vi "e.gate HighSpeedPort Diagnostics Internal.vi"(0 "e.gate Configuration":T1 {"StartTime" format="%#.10f"; "dActTimeToSecondFactor" format="%#.10f"; "StartTimeToDayFactor" format="%#_10f"}, 11 "error in (no error)":errorcluster) -> (4 "e.gate Configuration out":T1 {"StartTime" format="%#.10f"; "dActTimeToSecondFactor" format="%#.10f"; "StartTimeToDayFactor" format="%#_10f"}, 6 "e.gate Interface Diagnostic Data":T9={"Interface Kind"=["Fieldbus", "Internal System", "Internal System", "ExternalUART", "ExternalUART", "ExternalUART"], "Interface Index"=[0, 0, 0, 0, 1, 2], "Cycles Count"=[280401, 280401, 280401, 280401, 14024, 280401], "Error Count"=[0, 0, 0, 0, 0, 0], "DeltaTimeS"=[1402.004973, 1402.004982, 1402.004982, 1402.004982, 1402.004983, 1402.004983]}, 8 "e.gate Transport Diagnostic Data":T8, 10 "e.gate Variable Diagnostic Data":T7, 15 "error out":errorcluster)   [LabVIEW 2016]
uses:
  e.gate Diagnostic Interface Data.ctl
  e.gate Diagnostic Transport Data.ctl
  e.gate Diagnostic Variable Data.ctl
  e.gate Configuration.ctl
  e.gate Channel Data.ctl
  e.gate Data Type.ctl
  e.gate Protocol Type.ctl
  e.gate Module  Data.ctl
  e.gateHSP_DLLhandle.ctl
panel:
  out "Structure ID":i8
  out "Remaining Data":u8[](array[numeric])
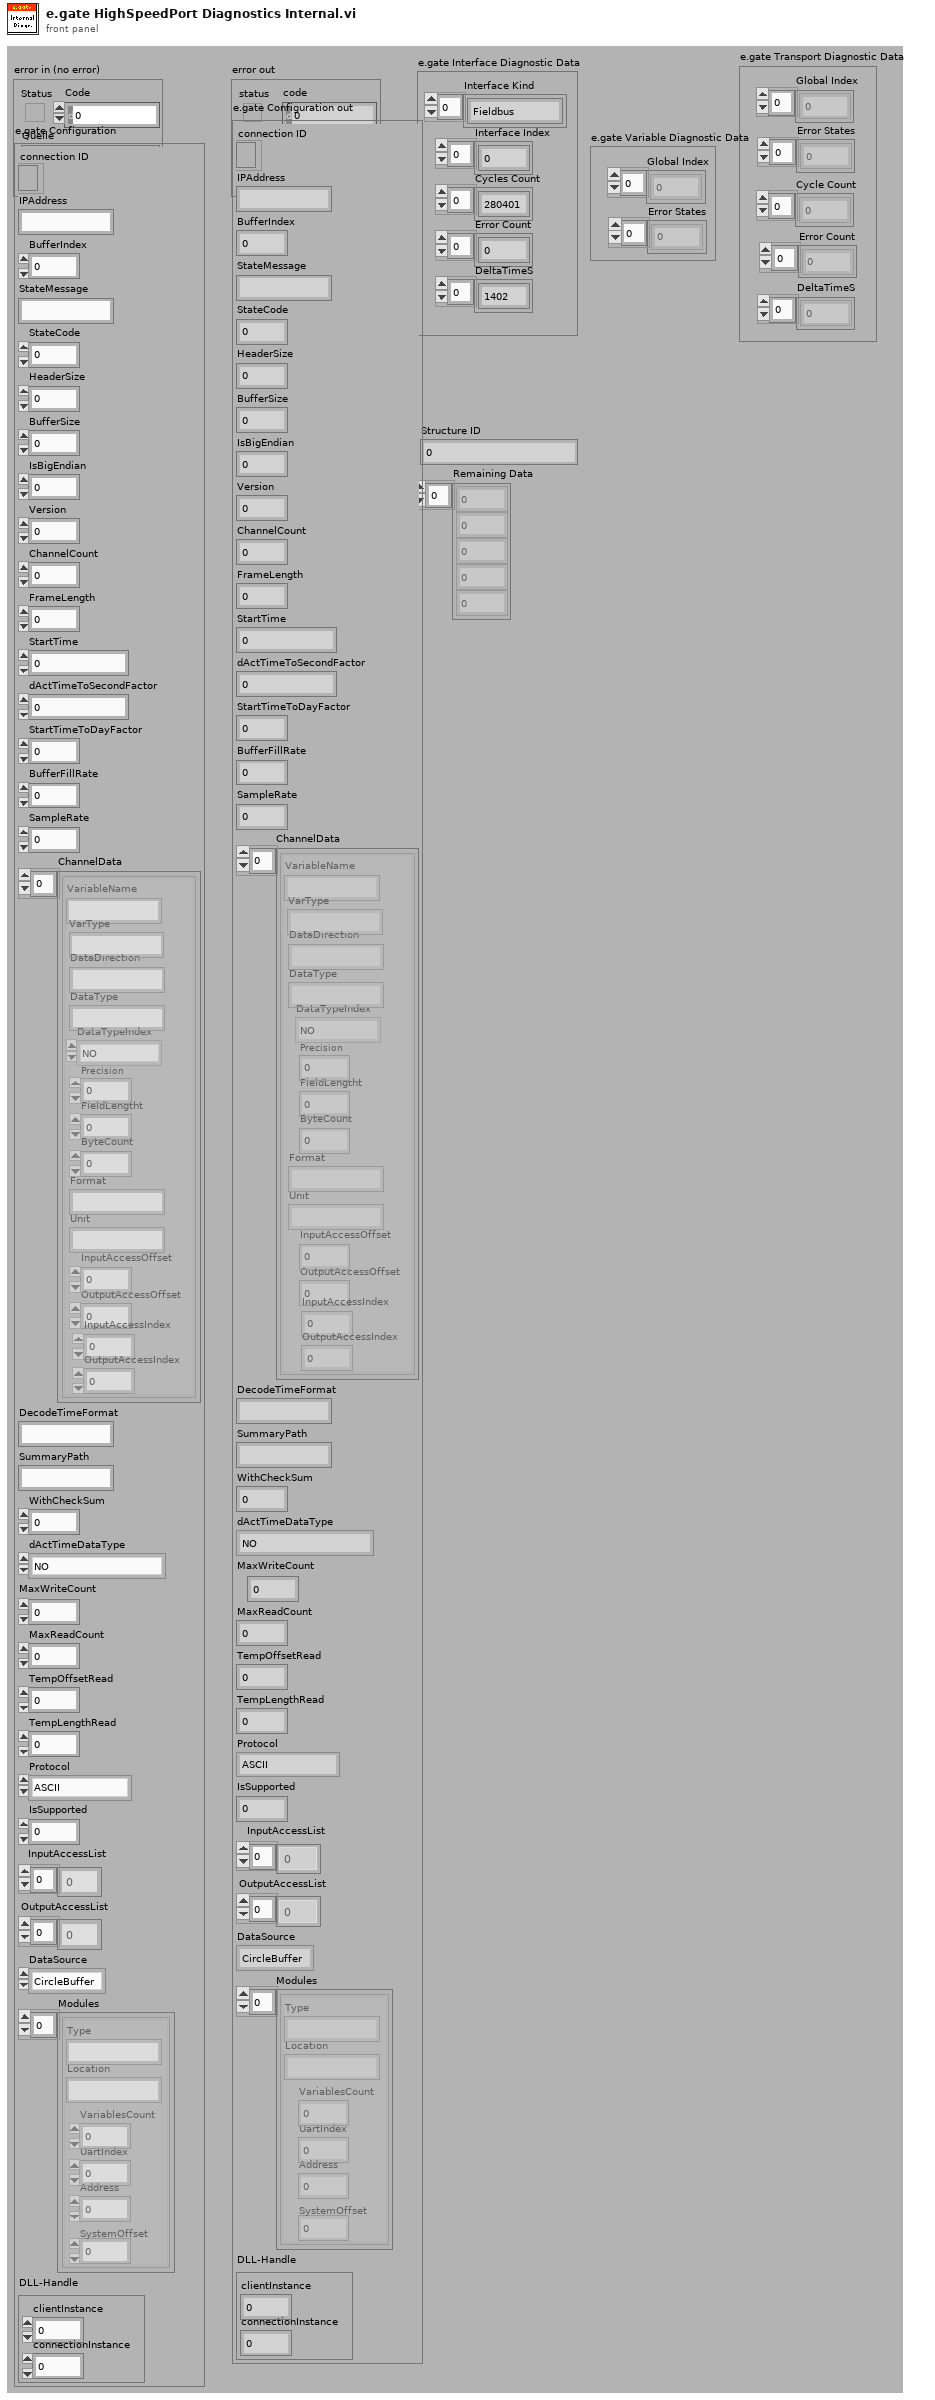
[diagram p1: front panel]
types:
  T1 = typedef "e.gate Configuration.ctl" = cluster{"connection ID":refnum<k5>, "IPAddress":string, "BufferIndex":i32, "StateMessage":string, "StateCode":i8, "HeaderSize":i32, "BufferSize":i32, "IsBigEndian":i32, "Version":i32, "ChannelCount":i32, "FrameLength":i32, "StartTime":dbl, "dActTimeToSecondFactor":dbl, "StartTimeToDayFactor":dbl, "BufferFillRate":dbl, "SampleRate":dbl, "ChannelData":T2[], "DecodeTimeFormat":string, "SummaryPath":string, "WithCheckSum":i32, "dActTimeDataType":T3, "MaxWriteCount":i32, "MaxReadCount":i32, "TempOffsetRead":i32, "TempLengthRead":i32, "Protocol":T4, "IsSupported":i32, "InputAccessList":i32[], "OutputAccessList":i32[], "DataSource":enum16{"CircleBuffer", "test.con Logger", "test.con Archive"}, "Modules":T5[], "DLL-Handle":T6}
  T2 = typedef "e.gate Channel Data.ctl" = cluster{"VariableName":string, "DataDirection":string, "DataType":string, "DataTypeIndex":T3, "Precision":i16, "FieldLengtht":i16, "ByteCount":i32, "Format":string, "Unit":string, "InputAccessOffset":i32, "OutputAccessOffset":i16, "InputAccessIndex":i16, "OutputAccessIndex":i16, "VarType":string}
  T3 = typedef "e.gate Data Type.ctl" = enum16{"NO", "BOOL", "SINT8", "USINT8", "SINT16", "USINT16", "SINT32", "USINT32", "FLOAT", "SET8", "SET16", "SET32", "DOUBLE", "SINT64", "USINT64", "SET64"}
  T4 = typedef "e.gate Protocol Type.ctl" = enum16{"ASCII", "HighspeedPort Online", "HighspeedPort Buffer", "eGateHighspeedPortDLL "}
  T5 = typedef "e.gate Module  Data.ctl" = cluster{"Type":string, "Location":string, "VariablesCount":i16, "UartIndex":i16, "Address":i16, "SystemOffset":i16}
  T6 = typedef "e.gateHSP_DLLhandle.ctl" = cluster{"clientInstance":i32, "connectionInstance":i32}
  T7 = typedef "e.gate Diagnostic Variable Data.ctl" = cluster{"Global Index":i16[], "Error States":i16[]}
  T8 = typedef "e.gate Diagnostic Transport Data.ctl" = cluster{"Global Index":i16[], "Error States":i16[], "Cycle Count":i32[], "Error Count":i32[], "DeltaTimeS":dbl[]}
  T9 = typedef "e.gate Diagnostic Interface Data.ctl" = cluster{"Interface Kind":string[], "Interface Index":i16[], "Cycles Count":i32[], "Error Count":i32[], "DeltaTimeS":dbl[]}
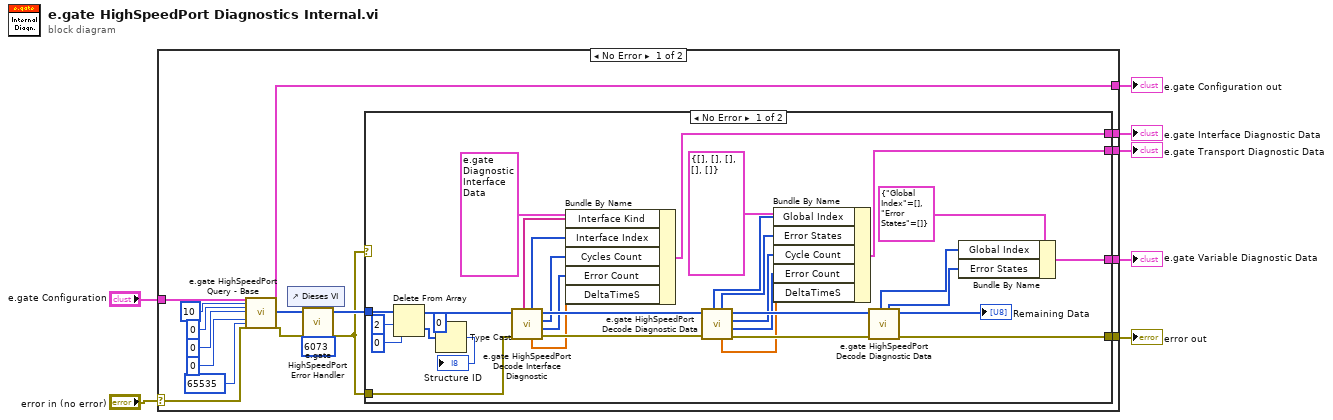
[diagram p0: block diagram]
diagram:
  n1 = case shown="No Error" "error in (no error)" {
    selector: "error in (no error)" -> [w20 w59]
    tunnel: "e.gate Configuration" -> [w25 w60]
    tunnel: [w18 w60] -> w4
    tunnel: [w17 w59] -> w3
    tunnel: [w16 _] -> w7
    tunnel: [w15 _] -> w6
    tunnel: [w14 _] -> w5
    frame No Error {
      n2 = call "e.gate HighSpeedPort Query - Base.vi"("e.gate Configuration in"=w25, "Command"=10, "OffsetWrite"=0, "LengthWrite"=0, "OffsetRead"=0, "LengthRead"=65535, "error in (no error)"=w20) -> ("e.gate Configuration out"=w18:T1, "Data (out binary)"=w11:u8[], "error out"=w10:errorcluster)  [unwired: 3 in, 15 out]
      n3 = control-ref of="Dieses VI"() -> (w13:refnum<vi>)
      n4 = call "e.gate HighSpeedPort Error Handler.vi"("error code start index"=6073, "VI reference"=w13, "error in (no error)"=w10, "binary data in"=w11) -> ("error out"=w8:errorcluster, "binary out"=w9:u8[])  [unwired: 6 out]
      n5 = case shown="No Error" w8 {
        tunnel: [w57 w58] -> w17
        tunnel: [w56 _] -> w16
        tunnel: [w55 _] -> w15
        tunnel: [w54 _] -> w14
        tunnel: w8 -> [w53 w58]
        tunnel: w9 -> [w52 _]
        frame No Error {
          n6 = Delete From Array(array=w52, length=2 ("Länge"), index=0 ("Index")) -> (deleted portion=w49:u8[], array with subset deleted=w46:u8[])
          n7 = Type Cast(type=i16 0, x=w49) -> (*(type *) &x=→"Structure ID":i16)
          n8 = call "e.gate HighSpeedPort Decode Interface Diagnostic.vi"("error in"=w53, "Binary Data in"=w46) -> ("error out"=w44:errorcluster, "Error Count"=w38:i32[], "Cycles Count"=w37:i32[], "Remaining Binary Data"=w45:u8[], "DeltaTimeS"=w39:dbl[], "Interface Index"=w36:i16[], "Interface Kind"=w35:string[])  [unwired: 1 in, 2 out]
          n9 = Bundle By Name(cluster=T9 {"Interface Kind"=["Fieldbus", "Internal System", "Internal System", "ExternalUART", "ExternalUART", "ExternalUART"], "Interface Index"=[0, 0, 0, 0, 1, 2], "Cycles Count"=[280401, 280401, 280401, 280401, 14024, 280401], "Error Count"=[0, 0, 0, 0, 0, 0], "DeltaTimeS"=[1402.004973, 1402.004982, 1402.004982, 1402.004982, 1402.004983, 1402.004983]} ("e.gate Interface Diagnostic Data"), "Interface Kind"=w35, "Interface Index"=w36, "Cycles Count"=w37, "Error Count"=w38, "DeltaTimeS"=w39) -> (w56:T9)
          n10 = call "e.gate HighSpeedPort Decode Diagnostic Data.vi"("error in"=w44, "Binary Data in"=w45) -> ("error out"=w42:errorcluster, "Error Count"=w32:i32[], "Cycle Count"=w31:i32[], "Remaining Binary Data"=w43:u8[], "DeltaTimeS"=w33:dbl[], "Error States"=w30:i16[], "Global Indexs"=w29:i16[])  [unwired: 1 in, 2 out]
          n11 = Bundle By Name(cluster=T8 {"Global Index"=[], "Error States"=[], "Cycle Count"=[], "Error Count"=[], "DeltaTimeS"=[]} ("e.gate Transport Diagnostic Data"), "Global Index"=w29, "Error States"=w30, "Cycle Count"=w31, "Error Count"=w32, "DeltaTimeS"=w33) -> (w55:T8)
          n12 = call "e.gate HighSpeedPort Decode Diagnostic Data.vi"("error in"=w42, "Binary Data in"=w43) -> ("error out"=w57:errorcluster, "Remaining Binary Data"=→"Remaining Data":u8[], "Error States"=w27:i16[], "Global Indexs"=w26:i16[])  [unwired: 1 in, 5 out]
          n13 = Bundle By Name(cluster=T7 {"Global Index"=[], "Error States"=[]} ("e.gate Variable Diagnostic Data"), "Global Index"=w26, "Error States"=w27) -> (w54:T7)
        }
        frame Error {
        }
      }
    }
    frame Error {
    }
  }
  "error out" <- w3
  "e.gate Interface Diagnostic Data" <- w7
  "e.gate Transport Diagnostic Data" <- w6
  "e.gate Variable Diagnostic Data" <- w5
  "e.gate Configuration out" <- w4
